vi "Character-H16.vi"(1 "string":string) -> (0 "string 2":string)   [LabVIEW 2019]
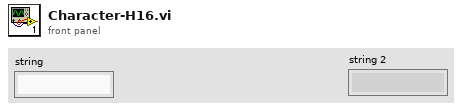
[diagram p1: front panel]
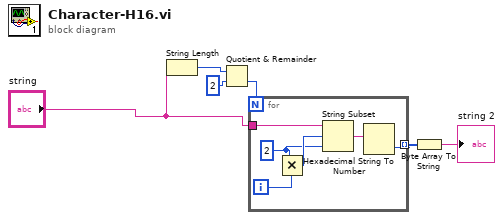
[diagram p0: block diagram]
diagram:
  n1 = String Length(string="string") -> (length=w5:i32)
  n2 = Quotient & Remainder(x=w5, y=2) -> (floor(x/y)=w6:i32)  [unwired: 1 out]
  n3 = for {
    N: w6 -> [_]
    tunnel: "string" -> [w9]
    tunnel: [w7] -> w3 mode=indexing
    i -> [w12]
    w10 = 2 ("y")
    n4 = Multiply(x=w10, y=w12) -> (x*y=w11:i32)
    n5 = String Subset(string=w9, offset (0)=w11, length (rest)=w10) -> (substring=w8:string)
    n6 = Hexadecimal String To Number(string=w8) -> (number=w7:u32)  [unwired: 2 in, 1 out]
  }
  n7 = Byte Array To String(unsigned byte array=w3) -> (string=→"string 2":string)
